vi "GetMeasurementTesting.vi"() -> ()   [LabVIEW 2012]
uses:
  <vilib>/LVH/i3 JSON/JSON Parsing/Get Object Parameter Files/Get Object Parameter - JSON Tree.vi
  <vilib>/LVH/i3 JSON/JSON Parsing/Get Object Parameter Files/Get Object Parameter - Numeric.vi
  <vilib>/LVH/i3 JSON/JSON Parsing/Get Object Parameter Files/Get Object Parameter - String.vi
  <vilib>/LVH/i3 JSON/i3-json.lvlib
  <vilib>/httpClient/LabVIEWHTTPClient.lvlib
panel:
  out "Array":T1(array[cluster])
  in  "padMeasurement":T2
  out "appended array":string[](array[string])
  out "variant out":variant
  in  "name":string
  out "Correponding data":i32
  out "Tree 4":string(tree)
  out "JSON Value (JSON Tree) 2":variant
  out "JSON Value (JSON Tree)":variant
  out "Tree 3":string(tree)
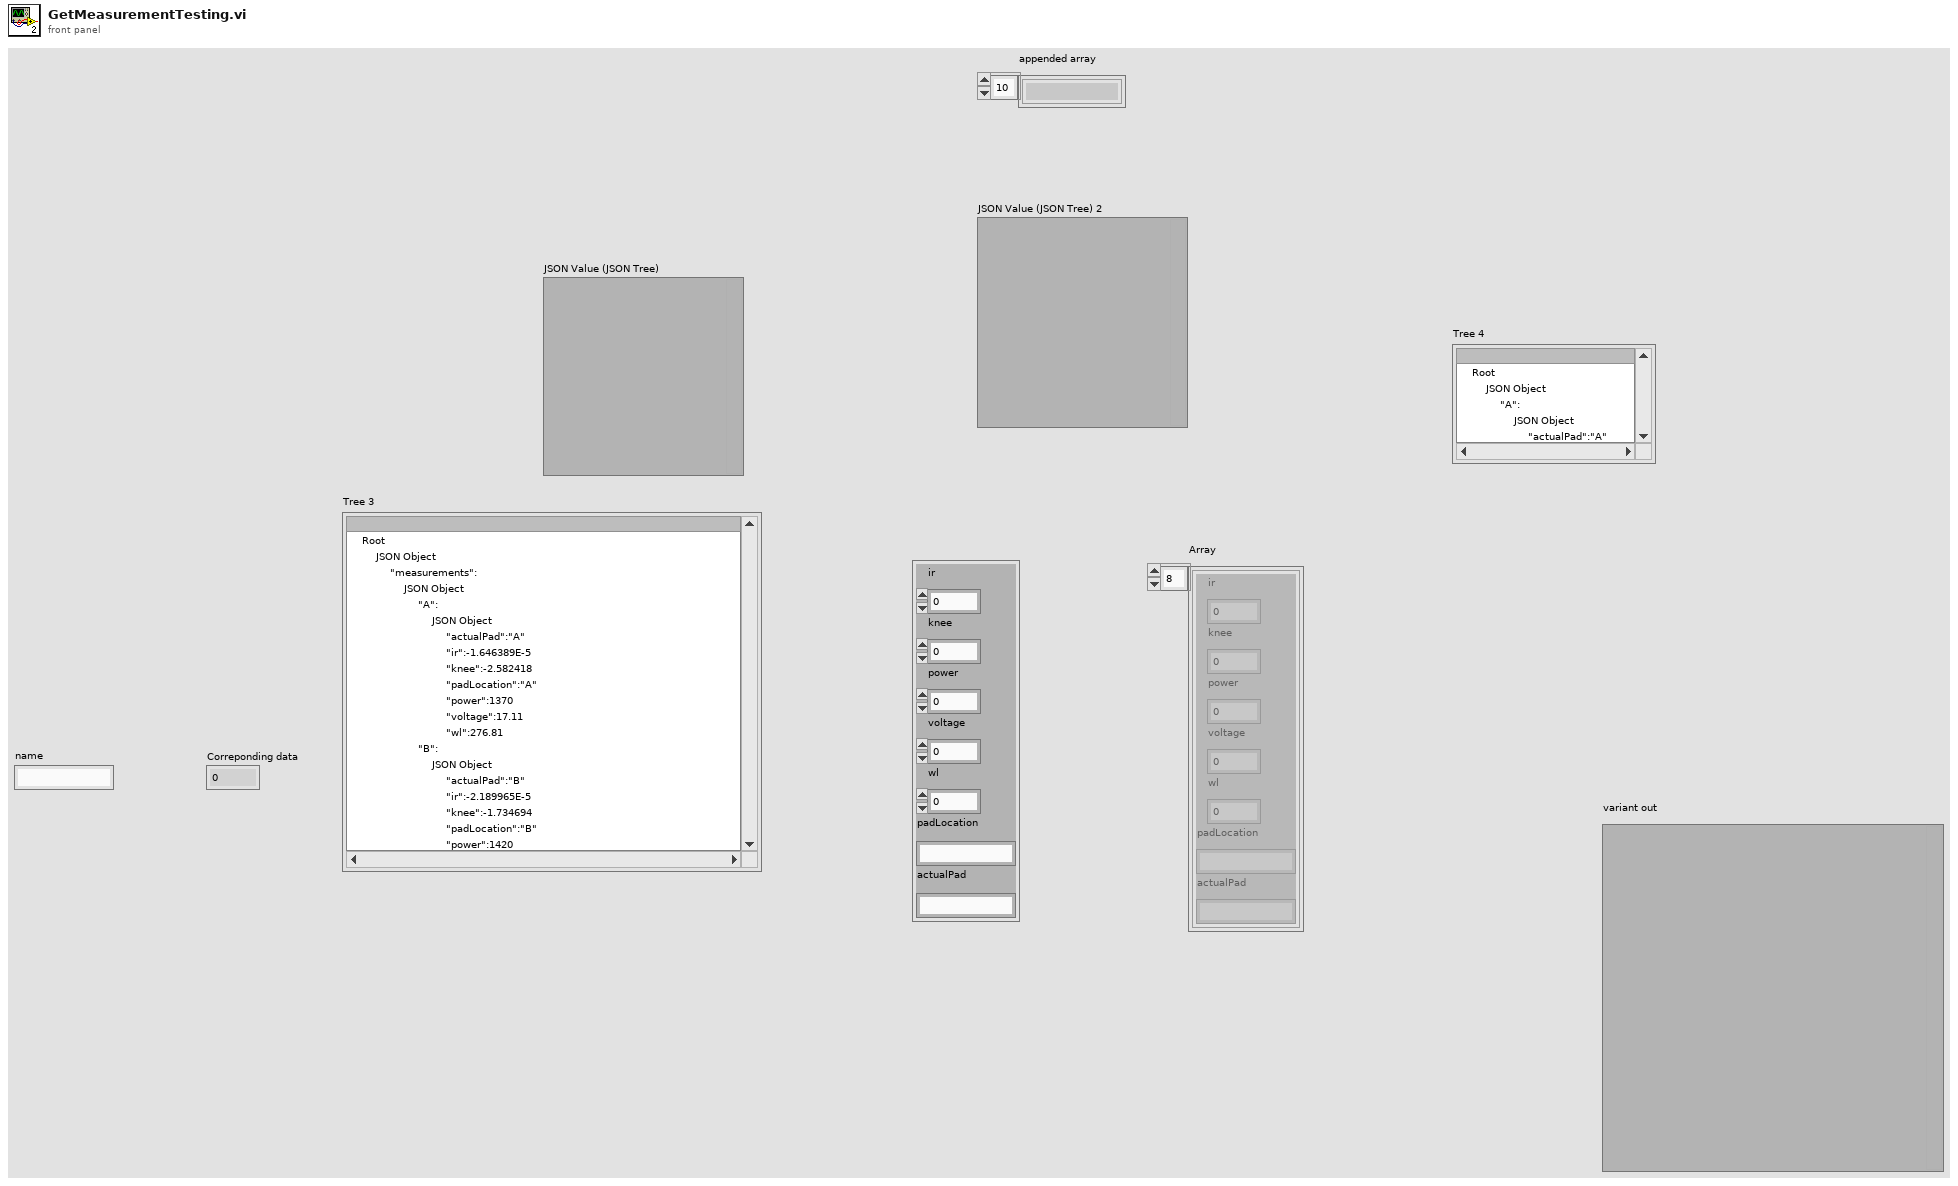
[diagram p1: front panel]
types:
  T1 = cluster{"ir":dbl, "knee":dbl, "power":dbl, "voltage":dbl, "wl":dbl, "padLocation":string, "actualPad":string}[]
  T2 = cluster{"ir":dbl, "knee":dbl, "power":dbl, "voltage":dbl, "wl":dbl, "padLocation":string, "actualPad":string}
  T3 = typedef "LabVIEWHTTPClient.lvlib/ClientHandle.ctl" = refnum<k1>
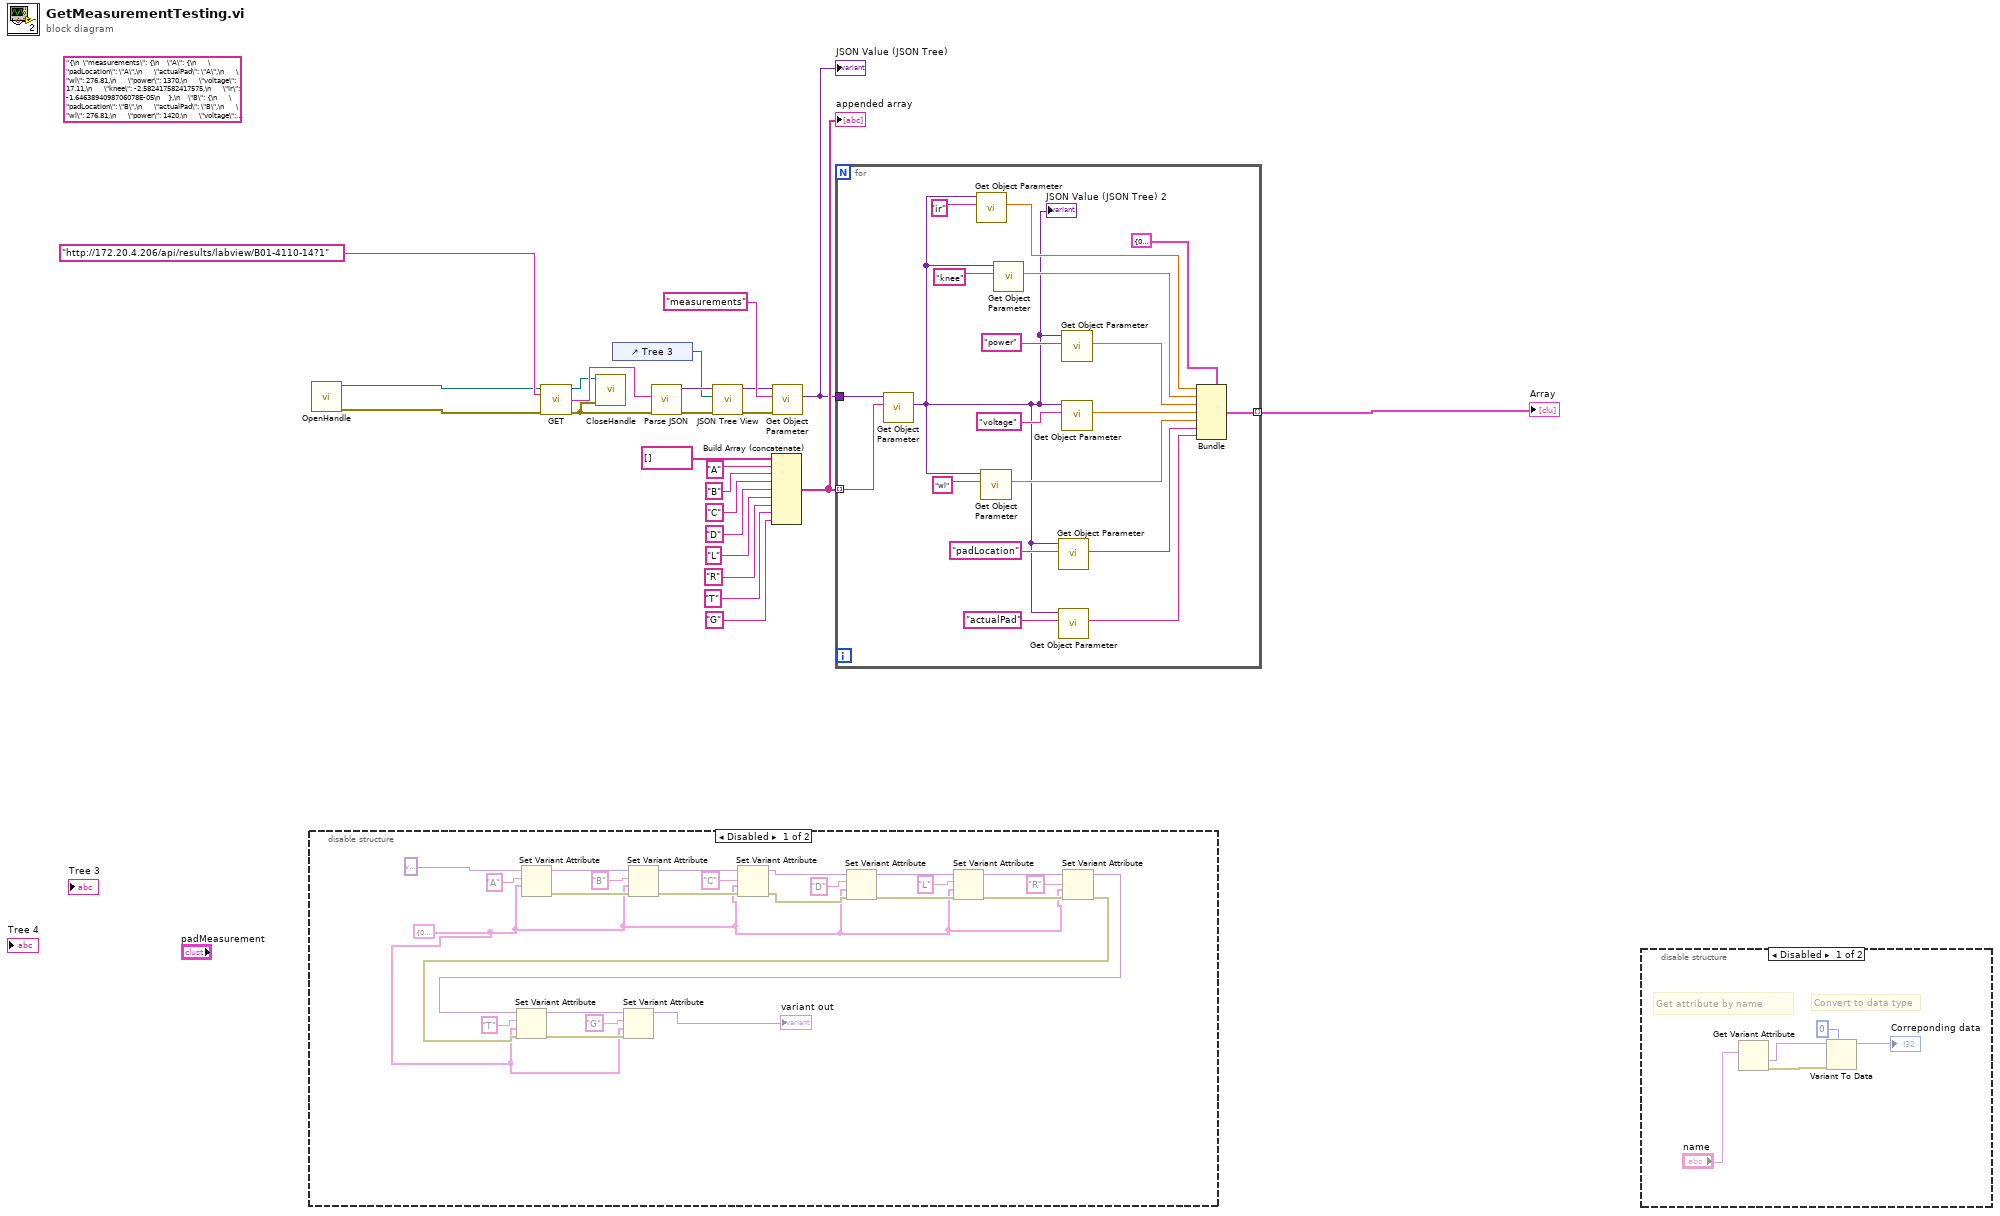
[diagram p0: block diagram]
diagram:
  (unwired) "{\n  \"measurements\": {\n    \"A\": {\n      \"padLocation\": \"A\",\n      \"actualPad\": \"A\",\n      \"wl\": 276.81,\n      \"power\": 1370,\n      \"voltage\": 17.11,\n      \"knee\": -2.582417582417575,\n      \"ir\": -1.6463894098706078E-05\n    },\n    \"B\": {\n      \"padLocation\": \"B\",\n      \"actualPad\": \"B\",\n      \"wl\": 276.81,\n      \"power\": 1420,\n      \"voltage\": 17.28,\n      \"knee\": -1.7346938775510032,\n      \"ir\": -2.189965234720148E-05\n    },\n    \"C\": {\n      \"padLocation\": \"C\",\n      \"actualPad\": \"\",\n      \"wl\": 0,\n      \"power\": 0,\n      \"voltage\": 0,\n      \"knee\": 0,\n      \"ir\": 0\n    },\n    \"D\": {\n      \"padLocation\": \"D\",\n      \"actualPad\": \"\",\n      \"wl\": 0,\n      \"power\": 0,\n      \"voltage\": 0,\n      \"knee\": 0,\n      \"ir\": 0\n    },\n    \"G\": {\n      \"padLocation\": \"G\",\n      \"actualPad\": \"G2-E\",\n      \"wl\": 272.69,\n      \"power\": 1180,\n      \"voltage\": 15.45,\n      \"knee\": -0.7017543859649122,\n      \"ir\": -1.9614652410382404E-05\n    },\n    \"L\": {\n      \"padLocation\": \"L\",\n      \"actualPad\": \"L2-E\",\n      \"wl\": 273.81,\n      \"power\": 1310,\n      \"voltage\": 18.7,\n      \"knee\": -1.712707182320442,\n      \"ir\": -1.8277976050740107E-05\n    },\n    \"R\": {\n      \"padLocation\": \"R\",\n      \"actualPad\": \"R2-E\",\n      \"wl\": 274.94,\n      \"power\": 1270,\n      \"voltage\": 18.69,\n      \"knee\": -1.16666666666666,\n      \"ir\": -1.6391380995628424E-05\n    },\n    \"T\": {\n      \"padLocation\": \"T\",\n      \"actualPad\": \"T2-E\",\n      \"wl\": 274.94,\n      \"power\": 1290,\n      \"voltage\": 19.78,\n      \"knee\": -2.1142857142856957,\n      \"ir\": -1.2373818026389927E-05\n    }\n  }\n}" ("JSON String")
  n1 = disable-structure shown="Disabled" {
    frame Disabled {
      w26 = T2 {"ir"=0.0, "knee"=0.0, "power"=0.0, "voltage"=0.0, "wl"=0.0, "padLocation"="", "actualPad"=""} ("padMeasurement")
      n2 = Set Variant Attribute(Variant=variant ("variant"), name="A", value=w26) -> (Variant out=w47:variant, error out=w46:errorcluster)  [unwired: 1 in, 1 out]
      n3 = Set Variant Attribute(Variant=w47, name="B", value=w26, error in=w46) -> (Variant out=w44:variant, error out=w43:errorcluster)  [unwired: 1 out]
      n4 = Set Variant Attribute(Variant=w44, name="C", value=w26, error in=w43) -> (Variant out=w30:variant, error out=w29:errorcluster)  [unwired: 1 out]
      n5 = Set Variant Attribute(Variant=w30, name="D", value=w26, error in=w29) -> (Variant out=w36:variant, error out=w37:errorcluster)  [unwired: 1 out]
      n6 = Set Variant Attribute(Variant=w36, name="L", value=w26, error in=w37) -> (Variant out=w39:variant, error out=w40:errorcluster)  [unwired: 1 out]
      n7 = Set Variant Attribute(Variant=w39, name="R", value=w26, error in=w40) -> (Variant out=w28:variant, error out=w27:errorcluster)  [unwired: 1 out]
      n8 = Set Variant Attribute(Variant=w28, name="T", value=w26, error in=w27) -> (Variant out=w33:variant, error out=w32:errorcluster)  [unwired: 1 out]
      n9 = Set Variant Attribute(Variant=w33, name="G", value=w26, error in=w32) -> (Variant out=→"variant out":variant)  [unwired: 2 out]
    }
    frame Enabled {
    }
  }
  n10 = call <vilib>:"OpenHandle.vi"() -> ("client handle out"=w13:T3, "error out"=w12:errorcluster)  [unwired: 14 in]
  n11 = call <vilib>:"GET.vi"("client handle"=w13, "url"="http://172.20.4.206/api/results/labview/B01-4110-14?1", "error in (no error)"=w12) -> ("client handle out"=w9:T3, "body"=w11:string, "error out"=w8:errorcluster)  [unwired: 9 in, 1 out]
  n12 = call <vilib>:"CloseHandle.vi"("client handle"=w9, "error in (no error)"=w8) -> ()  [unwired: 13 in, 1 out]
  n13 = control-ref of="Tree 3"() -> (w6:refnum<vi>)
  n14 = call <vilib>:"Parse JSON.vi"("error in (no error)"=w8, "JSON String"=w11) -> ("error out"=w7:errorcluster, "JSON Tree"=w10:variant)  [unwired: 6 in, 2 out]
  n15 = call <vilib>:"JSON Tree View.vi"("error in (no error)"=w7, "JSON Tree Expanded Reference"=w6, "JSON Tree"=w10) -> ("error out"=w4:errorcluster, "JSON Tree Passthrough"=w5:variant)  [unwired: 7 in]
  n16 = Build Array (concatenate)(string[] [], "A", "B", "C", "D", "L", "R", "T", "G") -> (w3:string[])
  "appended array" <- w3
  n17 = call-poly <vilib>:"Get Object Parameter.vi"("error in (no error)"=w4, "Parameter Name"="measurements", "JSON Tree In (JSON Object)"=w5) -> ("JSON Value (JSON Tree)"=w1:variant)  [unwired: 5 in, 3 out]
  "JSON Value (JSON Tree)" <- w1
  n18 = for {
    tunnel: w3 -> [w67] mode=indexing
    tunnel: w1 -> [w68]
    tunnel: [w50] -> w2 mode=indexing
    n19 = call-poly <vilib>:"Get Object Parameter.vi"("Parameter Name"=w67, "JSON Tree In (JSON Object)"=w68) -> ("JSON Value (JSON Tree)"=w53:variant)  [unwired: 6 in, 3 out]
    "JSON Value (JSON Tree) 2" <- w53
    n20 = call-poly <vilib>:"Get Object Parameter.vi"("Parameter Name"="ir", "JSON Tree In (JSON Object)"=w53) -> ("Double Value"=w64:dbl)  [unwired: 6 in, 3 out]
    n21 = call-poly <vilib>:"Get Object Parameter.vi"("Parameter Name"="wl", "JSON Tree In (JSON Object)"=w53) -> ("Double Value"=w60:dbl)  [unwired: 6 in, 3 out]
    n22 = call-poly <vilib>:"Get Object Parameter.vi"("Parameter Name"="knee", "JSON Tree In (JSON Object)"=w53) -> ("Double Value"=w63:dbl)  [unwired: 6 in, 3 out]
    n23 = call-poly <vilib>:"Get Object Parameter.vi"("Parameter Name"="padLocation", "JSON Tree In (JSON Object)"=w53) -> ("String Value"=w51:string)  [unwired: 6 in, 3 out]
    n24 = call-poly <vilib>:"Get Object Parameter.vi"("Parameter Name"="actualPad", "JSON Tree In (JSON Object)"=w53) -> ("String Value"=w52:string)  [unwired: 6 in, 3 out]
    n25 = call-poly <vilib>:"Get Object Parameter.vi"("Parameter Name"="power", "JSON Tree In (JSON Object)"=w53) -> ("Double Value"=w62:dbl)  [unwired: 6 in, 3 out]
    n26 = call-poly <vilib>:"Get Object Parameter.vi"("Parameter Name"="voltage", "JSON Tree In (JSON Object)"=w53) -> ("Double Value"=w61:dbl)  [unwired: 6 in, 3 out]
    n27 = Bundle(cluster=T2 {"ir"=0.0, "knee"=0.0, "power"=0.0, "voltage"=0.0, "wl"=0.0, "padLocation"="", "actualPad"=""} ("padMeasurement"), "ir"=w64, "knee"=w63, "power"=w62, "voltage"=w61, "wl"=w60, "padLocation"=w51, "actualPad"=w52) -> (w50:T2)
  }
  "Array" <- w2
  n28 = disable-structure shown="Disabled" {
    frame Disabled {
      # "Convert to data type"
      # "Get attribute by name"
      n29 = Get Variant Attribute(name="name") -> (value=w73:variant, error out=w72:errorcluster)  [unwired: 3 in, 2 out]
      n30 = Variant To Data(error in=w72, type=0, Variant=w73) -> (data=→"Correponding data":i32)  [unwired: 1 out]
    }
    frame Enabled {
    }
  }
